vi "Example_Sys_ID.vi"() -> ()   [LabVIEW 2020]
uses:
  <vilib>/Analysis/Matrix/Datatypes/RealMatrix.ctl
  <vilib>/Analysis/Matrix/NI_Matrix.lvlib
panel:
  out "Right Motor Output":dbl(graph)
  in  "Input Order":i32=1
  in  "Output Order":i32=2
  out "RMSE":dbl format="%0.2f"
  out "Output vs Model":dbl[][](graph)
  out "Resultant Parameters\nOutput-Input":T1
  out "Right Motor Input":dbl(graph)
  out "SonarDistance":dbl
  in  "ServoAngle":dbl
  in  "ControlR (-1 to 1)":dbl
  in  "IP Address":string="192.168.1.1"
  in  "Mode Select":T2(ring)
  out "Velocity Right":dbl
  out "Velocity Left":dbl
  in  "dt (ms)":u32=10
  in  "ControlL (-1 to 1)":dbl min=-1.0 max=1.0 step=0.01
  in  "Stop":bool
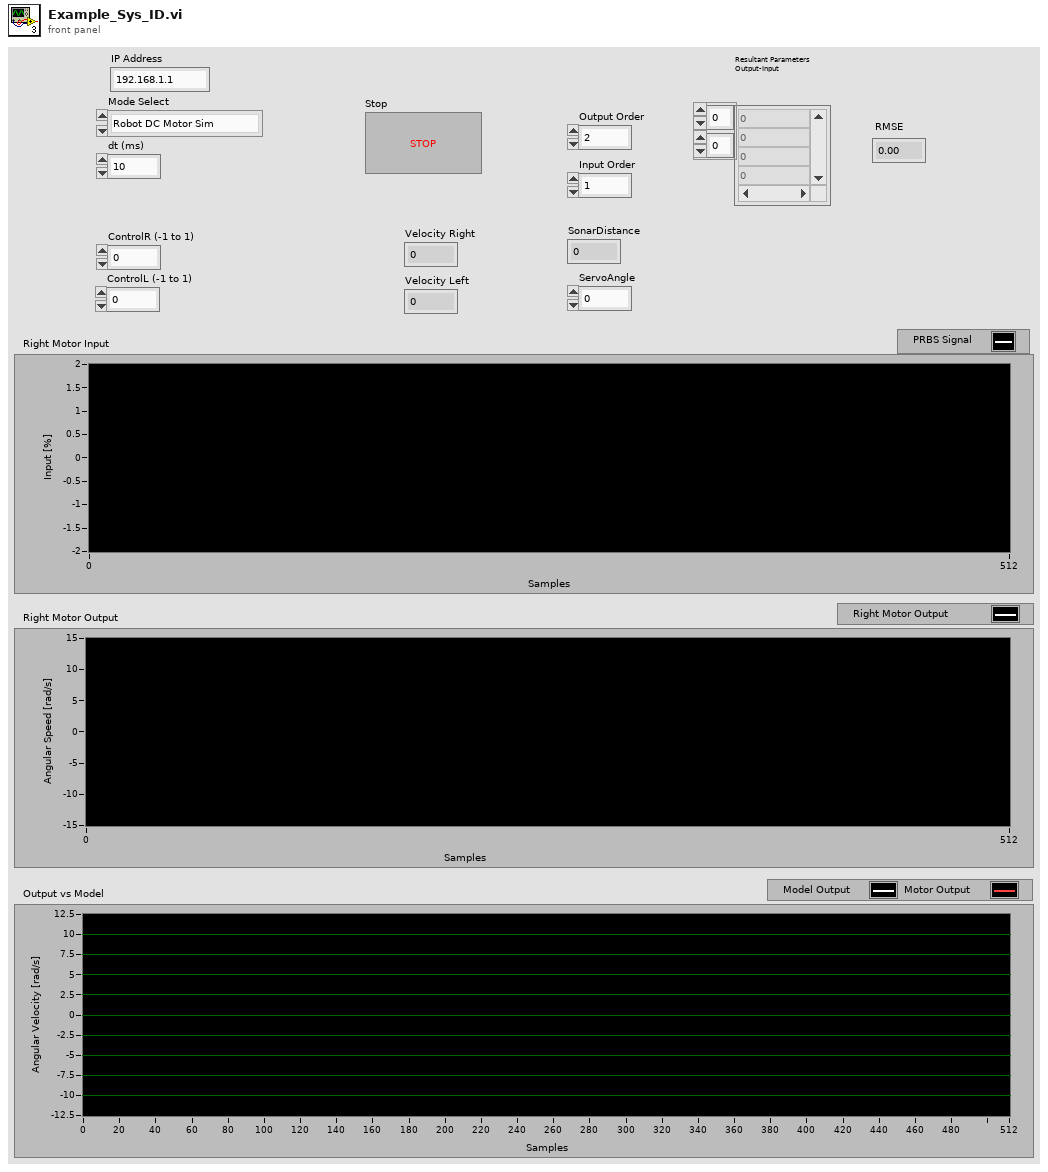
[diagram p1: front panel]
types:
  T1 = typedef "NI_Matrix.lvlib/RealMatrix.ctl" = dbl[][]
  T2 = enum16{"Robot DC Motor Sim", "Robot Simulation", "Real Robot"}
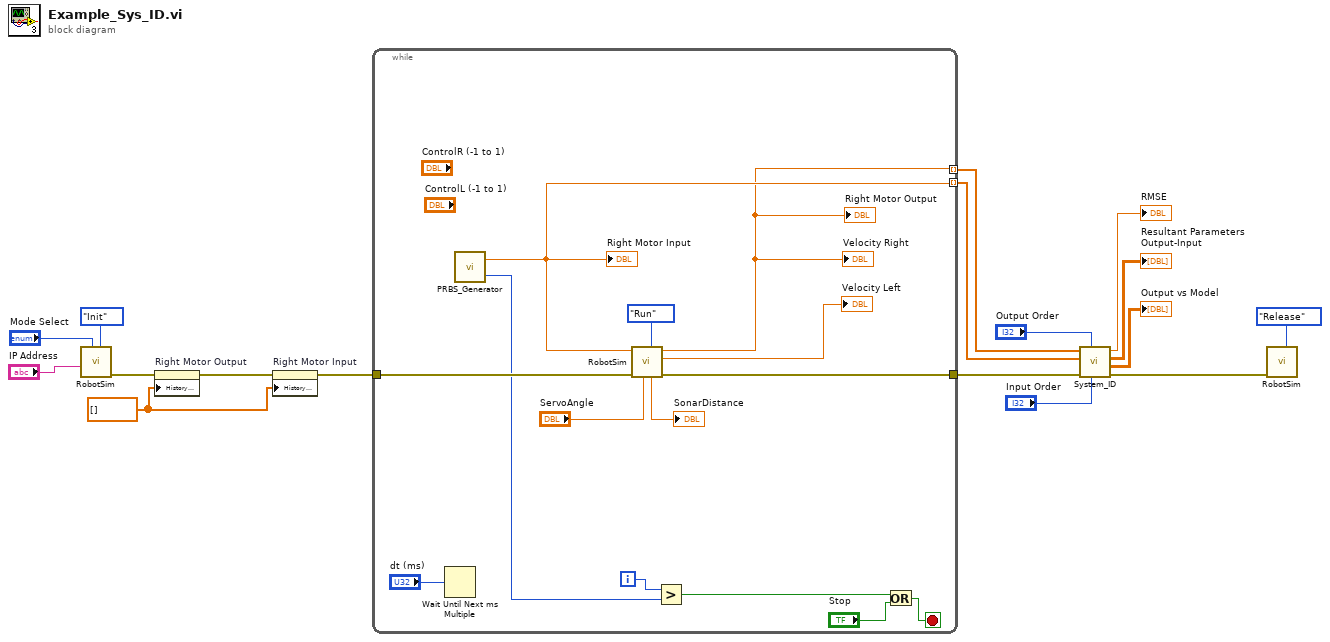
[diagram p0: block diagram]
diagram:
  w1 = dbl[] [] ("History Data")
  n1 = call "RobotSim.vi"("Action"=enum16{"Init", "Run", "Release"}."Init", "Mode Select"="Mode Select", "IP Address"="IP Address") -> ("error out"=w2:errorcluster)  [unwired: 4 in, 4 out]
  n2 = property on="Right Motor Output" class="WFChart (strict)"(error in=w2, "History Data"=w1) -> (error out=w3:errorcluster)  [unwired: 1 in, 1 out]
  n3 = property on="Right Motor Input" class="WFChart (strict)"(error in=w3, "History Data"=w1) -> (error out=w13:errorcluster)  [unwired: 1 in, 1 out]
  n4 = while {
    tunnel: w13 -> [w30]
    tunnel: [w28] -> w5
    tunnel: [w18] -> w7 mode=indexing
    tunnel: [w19] -> w6 mode=indexing
    i -> [w25]
    stop <- w20 stop-if-true
    n5 = Wait Until Next ms Multiple(millisecond multiple="dt (ms)") -> ()  [unwired: 1 out]
    n6 = call "PRBS_Generator.vi"() -> ("Size"=w23:i32, "PRBS Output"=w19:dbl)  [unwired: 2 in]
    "Right Motor Input" <- w19
    n7 = call "RobotSim.vi"("Action"=enum16{"Init", "Run", "Release"}."Run", "ServoAngle"="ServoAngle", "error in (no error)"=w30, "ControlR"=w19) -> ("error out"=w28:errorcluster, "OmegaL"=→"Velocity Left":dbl, "OmegaR"=w18:dbl, "SonarDistance"=→"SonarDistance":dbl)  [unwired: 3 in, 1 out]
    "Velocity Right" <- w18
    "Right Motor Output" <- w18
    n8 = Greater?(x=w25, y=w23) -> (0:w21:bool)
    n9 = Or(x=w21, y="Stop") -> (x .or. y?=w20:bool)
  }
  n10 = call "System_ID.vi"("Input Order"="Input Order", "Output Order"="Output Order", "error in (no error)"=w5, "Input Array"=w6, "Output Array"=w7) -> ("error out"=w4:errorcluster, "Output vs Model"=→"Output vs Model":dbl[][], "Resultant Parameters"=→"Resultant Parameters\nOutput-Input":T1, "RMSE"=→"RMSE":dbl)  [unwired: 1 in]
  n11 = call "RobotSim.vi"("Action"=enum16{"Init", "Run", "Release"}."Release", "error in (no error)"=w4) -> ()  [unwired: 5 in, 5 out]
